vi "ErrorDialog.vi"(8 "error in (no error)":errorcluster, 11 "message":string) -> ()   [LabVIEW 2013]
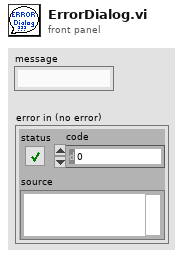
[diagram p1: front panel]
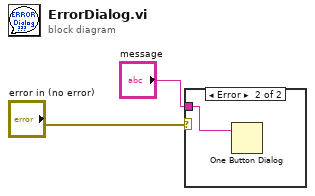
[diagram p0: block diagram]
diagram:
  n1 = case shown="Error" "error in (no error)" {
    tunnel: "message" -> [_ w3]
    frame No Error {
    }
    frame Error {
      n2 = One Button Dialog(message=w3) -> ()  [unwired: 1 in, 1 out]
    }
  }
